vi "Grow Snake.vi"(11 "Snake in":refnum<class "Snake.lvclass">) -> ()   [LabVIEW 2021, in "Snake.lvclass"]
uses:
  Snake.lvclass
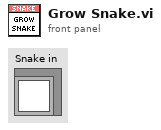
[diagram p1: front panel]
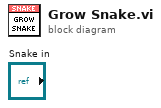
[diagram p0: block diagram]
diagram:
